vi "__ExpandNameMapIfNeeded.vi"(9 "Numeric":i32, 11 "NameMap A in":T1) -> (3 "NameMap A out":T1)   [LabVIEW 2019, in "lv-apt-json-file.lvlib"]
uses:
  Typedef/Def-NameMap.ctl
  lv-apt-json-file.lvlib
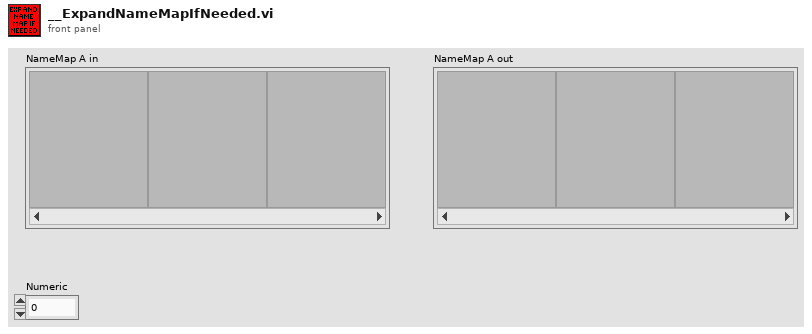
[diagram p1: front panel]
types:
  T1 = typedef "lv-apt-json-file.lvlib/Def-NameMap.ctl" = variant[]
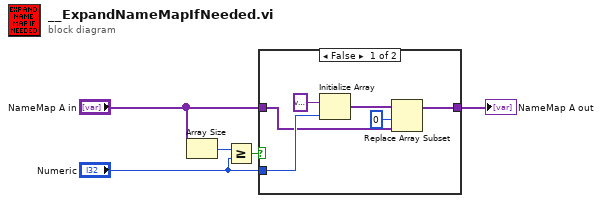
[diagram p0: block diagram]
diagram:
  n1 = Array Size(array="NameMap A in") -> (size(s)=w2:i32)
  n2 = Greater Or Equal?(x=w2, y="Numeric") -> (x >= y?=w1:bool)
  n3 = case shown="False" w1 {
    tunnel: "NameMap A in" -> [w8 w12]
    tunnel: [w6 w12] -> w5
    tunnel: "Numeric" -> [w11 _]
    frame False {
      n4 = Initialize Array(variant, w11) -> (w9:variant[])
      n5 = Replace Array Subset(array=w9, new element=w8, index=0) -> (w6:variant[])
    }
    frame True {
    }
  }
  "NameMap A out" <- w5
